vi "String.Font size to Pixel Height.vi"(11 "Font":i16) -> (3 "Pixel Height":i16)   [LabVIEW 2018]
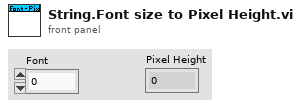
[diagram p1: front panel]
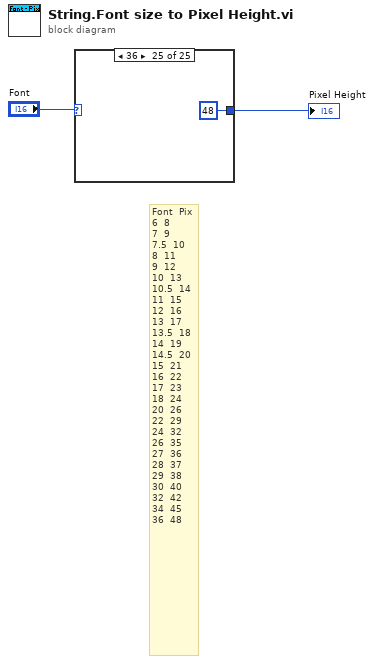
[diagram p0: block diagram]
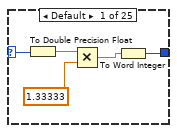
[diagram p2: hidden frame]
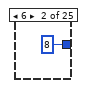
[diagram p3: hidden frame]
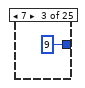
[diagram p4: hidden frame]
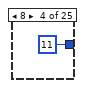
[diagram p5: hidden frame]
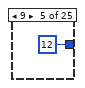
[diagram p6: hidden frame]
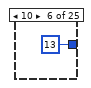
[diagram p7: hidden frame]
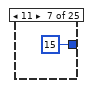
[diagram p8: hidden frame]
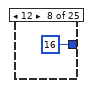
[diagram p9: hidden frame]
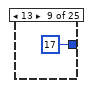
[diagram p10: hidden frame]
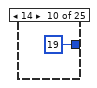
[diagram p11: hidden frame]
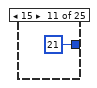
[diagram p12: hidden frame]
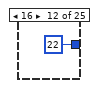
[diagram p13: hidden frame]
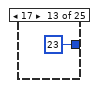
[diagram p14: hidden frame]
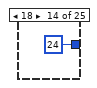
[diagram p15: hidden frame]
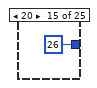
[diagram p16: hidden frame]
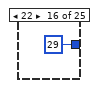
[diagram p17: hidden frame]
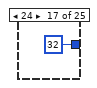
[diagram p18: hidden frame]
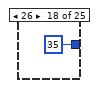
[diagram p19: hidden frame]
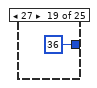
[diagram p20: hidden frame]
diagram:
  # "Font\t\tPix\n6\t\t8\n7\t\t9\n7.5\t\t10\n8\t\t11\n9\t\t12\n10\t\t13\n10.5\t\t14\n11\t\t15\n12\t\t16\n13\t\t17\n13.5\t\t18\n14\t\t19\n14.5\t\t20\n15\t\t21\n16\t\t22\n17\t\t23\n18\t\t24\n20\t\t26\n22\t\t29\n24\t\t32\n26\t\t35\n27\t\t36\n28\t\t37\n29\t\t38\n30\t\t40\n32\t\t42\n34\t\t45\n36\t\t48"
  n1 = case shown="36" "Font" {
    selector: "Font" -> [w7 _ _ _ _ _ _ _ _ _ _ _ _ _ _ _ _ _ _ _ _ _ _ _ _]
    tunnel: [w4 i16 8 i16 9 i16 11 i16 12 i16 13 i16 15 i16 16 i16 17 i16 19 i16 21 i16 22 i16 23 i16 24 i16 26 i16 29 i16 32 i16 35 i16 36 i16 37 i16 38 i16 40 i16 42 i16 45 i16 48] -> w1
    frame Default {
      n2 = To Double Precision Float(number=w7) -> (double precision float=w6:dbl)
      n3 = Multiply(x=w6, y=1.33333) -> (x*y=w3:dbl)
      n4 = To Word Integer(number=w3) -> (16bit integer=w4:i16)
    }
    frame 6 {
    }
    frame 7 {
    }
    frame 8 {
    }
    frame 9 {
    }
    frame 10 {
    }
    frame 11 {
    }
    frame 12 {
    }
    frame 13 {
    }
    frame 14 {
    }
    frame 15 {
    }
    frame 16 {
    }
    frame 17 {
    }
    frame 18 {
    }
    frame 20 {
    }
    frame 22 {
    }
    frame 24 {
    }
    frame 26 {
    }
    frame 27 {
    }
    frame 28 {
    }
    frame 29 {
    }
    frame 30 {
    }
    frame 31 {
    }
    frame 34 {
    }
    frame 36 {
    }
  }
  "Pixel Height" <- w1
